vi "Filter Duplicate Images out.vi"(8 "Error In":errorcluster, 9 "GreyLevel Drops and time Derivative in":dbl[][](array[numeric]), 10 "GreyLevel Drops and time in":dbl[][](array[numeric]), 11 "Rel Time (s) in":u32[](array[numeric])) -> (0 "Error Out":errorcluster, 1 "GreyLevel Drops and time Derivative out":dbl[][](array[numeric]), 2 "GreyLevel Drops and time out":dbl[][](array[numeric]), 3 "Rel Time (s) out":u32[](array[numeric]))   [LabVIEW 2015]
panel:
  # "Filters Duplicate images by checking when the derivative is zero"
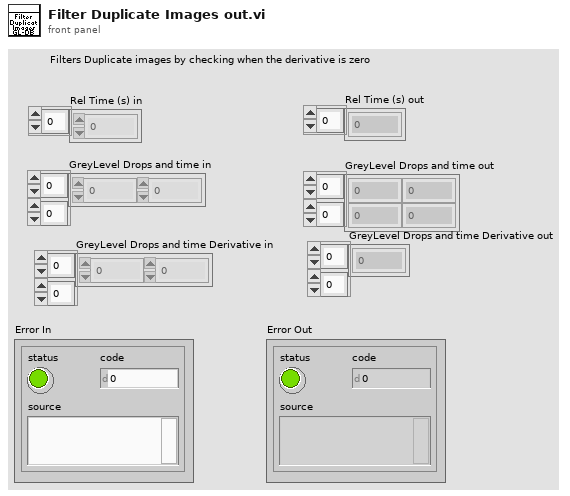
[diagram p1: front panel]
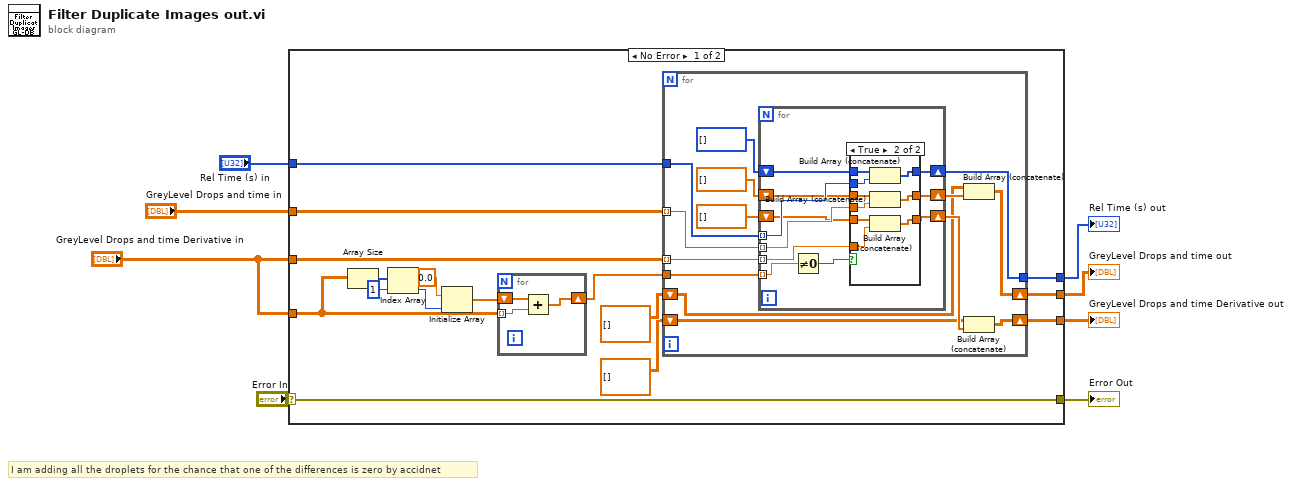
[diagram p0: block diagram]
diagram:
  # "I am adding all the droplets for the chance that one of the differences is zero by accidnet"
  n1 = case shown="No Error" "Error In" {
    selector: "Error In" -> [w24 w68]
    tunnel: [w24 w68] -> w7
    tunnel: [w17 w67] -> w6
    tunnel: "Rel Time (s) in" -> [w23 w67]
    tunnel: [w21 w66] -> w4
    tunnel: "GreyLevel Drops and time in" -> [w22 w66]
    tunnel: [w20 w65] -> w2
    tunnel: "GreyLevel Drops and time Derivative in" -> [w16 w65]
    tunnel: "GreyLevel Drops and time Derivative in" -> [w12 _]
    frame No Error {
      n2 = Array Size(array=w12) -> (size(s)=w11:i32[])
      n3 = Index Array(array=w11, index=1) -> (element=w10:i32)
      n4 = Initialize Array(0.0 ("element"), w10) -> (w9:dbl[])
      n5 = for {
        tunnel: w12 -> [w27] mode=indexing
        shift-right: [w26] -> w15
        shift-left: w9 -> [w25]
        n6 = Add(x=w25, y=w27) -> (x+y=w26:dbl[])
      }
      n7 = for {
        tunnel: w23 -> [w40]
        tunnel: w22 -> [w41] mode=indexing
        tunnel: w16 -> [w29] mode=indexing
        shift-right: [w36] -> w21
        shift-left: dbl[][] [] -> [w35]
        shift-right: [w37] -> w20
        shift-left: dbl[][] [] -> [w34]
        tunnel: [w30] -> w17
        tunnel: w15 -> [w28]
        n8 = for {
          tunnel: w29 -> [w52] mode=indexing
          tunnel: w41 -> [w51] mode=indexing
          tunnel: w40 -> [w50] mode=indexing
          shift-right: [w49] -> w30
          shift-left: u32[] [] -> [w48]
          shift-right: [w46] -> w38
          shift-left: dbl[] [] -> [w44]
          shift-right: [w47] -> w39
          shift-left: dbl[] [] -> [w45]
          tunnel: w28 -> [w42] mode=indexing
          n9 = Not Equal To 0?(x=w42) -> (x != 0?=w43:bool)
          n10 = case shown="True" w43 {
            tunnel: w52 -> [_ w64]
            tunnel: w51 -> [_ w63]
            tunnel: w50 -> [_ w62]
            tunnel: [w55 w61] -> w49
            tunnel: w48 -> [w55 w60]
            tunnel: [w54 w59] -> w47
            tunnel: [w53 w58] -> w46
            tunnel: w45 -> [w54 w57]
            tunnel: w44 -> [w53 w56]
            frame False {
            }
            frame True {
              n11 = Build Array (concatenate)(w60, w62) -> (w61:u32[])
              n12 = Build Array (concatenate)(w57, w63) -> (w59:dbl[])
              n13 = Build Array (concatenate)(w56, w64) -> (w58:dbl[])
            }
          }
        }
        n14 = Build Array (concatenate)(w35, w39) -> (w36:dbl[][])
        n15 = Build Array (concatenate)(w34, w38) -> (w37:dbl[][])
      }
    }
    frame Error {
    }
  }
  "Error Out" <- w7
  "Rel Time (s) out" <- w6
  "GreyLevel Drops and time out" <- w4
  "GreyLevel Drops and time Derivative out" <- w2
